vi "bedingungen editor.vi"() -> ()   [LabVIEW 2010]
panel:
  in  "Abfrage Nummer":u32
  in  "löschen":bool
  out "Array":string[][](array[string])
  in  "Stopp":bool
  in  "Abfrage übernehmen":bool
  in  "WertC\n---------------------\nSchreibweise: 0,0042\nT=True; F=False":string
  in  "VariableC":string(combo)
  in  "WertA\n---------------------\nSchreibweise: 0,0042\nT=True; F=False\n---=ungültig":string
  in  "VariableB":string(combo)
  in  "Vergleichsoperator":string(combo)
  in  "VariableA":string(combo)
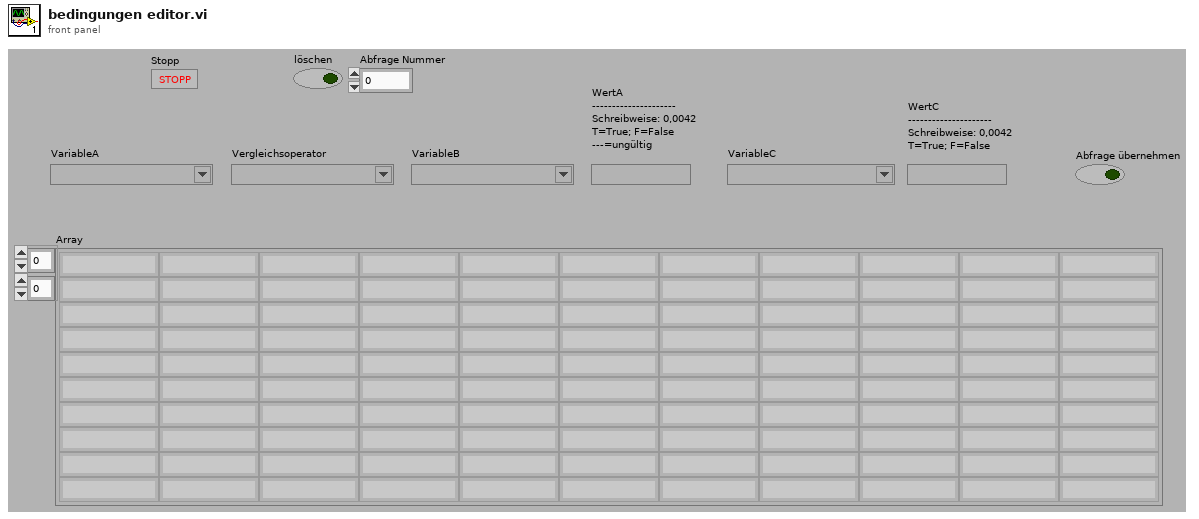
[diagram p1: front panel]
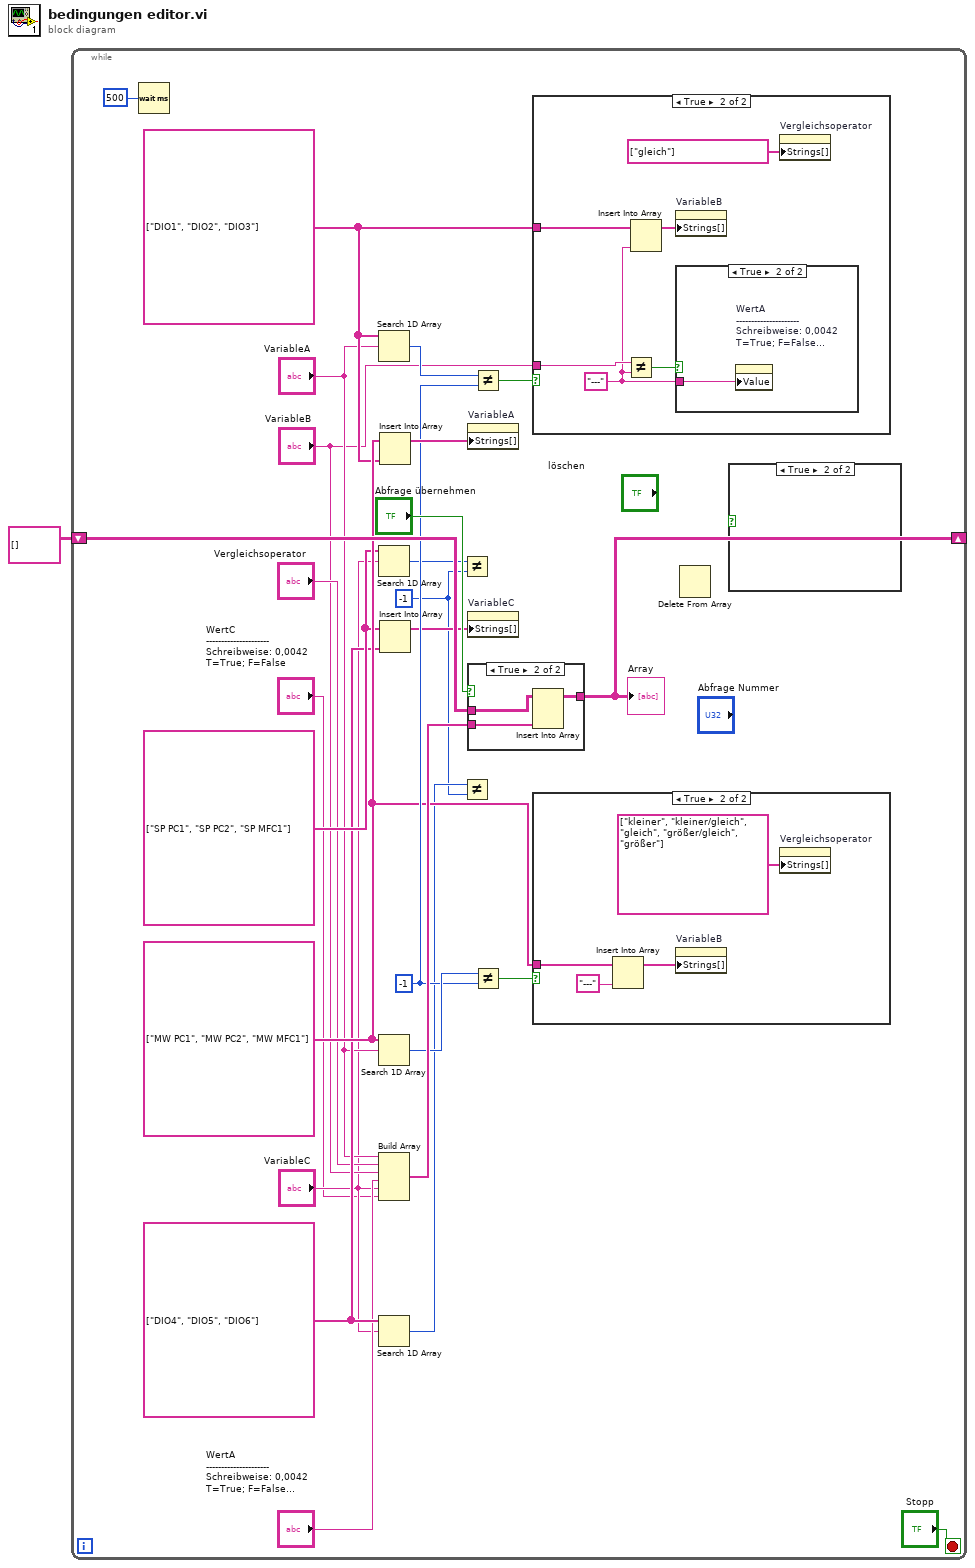
[diagram p0: block diagram]
diagram:
  n1 = while {
    shift-right: [w23] -> _
    shift-left: string[][] [] -> [w24]
    stop <- "Stopp" stop-if-true
    w8 = -1 ("y")
    w10 = string[] ["DIO4", "DIO5", "DIO6"] ("Strings []")
    w12 = string[] ["SP PC1", "SP PC2", "SP MFC1"] ("Strings []")
    w18 = -1 ("y")
    w14 = string[] ["DIO1", "DIO2", "DIO3"] ("Strings []")
    w15 = string[] ["MW PC1", "MW PC2", "MW MFC1"] ("Strings []")
    n2 = Wait (ms)(milliseconds to wait=u32 500 ("Zu wartende ms")) -> ()  [unwired: 1 out]
    n3 = Search 1D Array(1D array=w14, element="VariableA") -> (index of element=w19:i32)  [unwired: 1 in]
    n4 = Search 1D Array(1D array=w12, element="VariableC") -> (index of element=w11:i32)  [unwired: 1 in]
    n5 = Search 1D Array(1D array=w15, element="VariableA") -> (index of element=w20:i32)  [unwired: 1 in]
    n6 = Build Array("VariableA", "Vergleichsoperator", "VariableB", "WertA\n---------------------\nSchreibweise: 0,0042\nT=True; F=False\n---=ungültig", "VariableC", "WertC\n---------------------\nSchreibweise: 0,0042\nT=True; F=False") -> (w25:string[])
    n7 = Search 1D Array(1D array=w10, element="VariableC") -> (index of element=w9:i32)  [unwired: 1 in]
    n8 = Insert Into Array(array=w15, new element=w14) -> (w21:string[])  [unwired: 1 in]
    n9 = Insert Into Array(array=w12, new element=w10) -> (w13:string[])  [unwired: 1 in]
    n10 = Not Equal?(x=w11, y=w8) -> ()  [unwired: 1 out]
    n11 = Not Equal?(x=w9, y=w8) -> ()  [unwired: 1 out]
    n12 = property on="VariableA" class="KombiFeld"("Strings[]"=w21) -> ()  [unwired: 2 in, 2 out]
    n13 = property on="VariableC" class="KombiFeld"("Strings[]"=w13) -> ()  [unwired: 2 in, 2 out]
    n14 = case shown="True" "Abfrage übernehmen" {
      tunnel: w25 -> [_ w41]
      tunnel: w24 -> [w39 w42]
      tunnel: [w39 w40] -> w23
      frame False {
      }
      frame True {
        n15 = Insert Into Array(array=w42, new element=w41) -> (w40:string[][])  [unwired: 2 in]
      }
    }
    "Array" <- w23
    n16 = Not Equal?(x=w19, y=w18) -> (x != y?=w16:bool)
    n17 = Not Equal?(x=w20, y=w18) -> (x != y?=w17:bool)
    n18 = case shown="True" w16 {
      tunnel: w14 -> [_ w32]
      tunnel: "VariableB" -> [_ w30]
      frame False {
      }
      frame True {
        w28 = "---" ("Neues Element/Teil-Array")
        n19 = Not Equal?(x=w30, y=w28) -> (x != y?=w29:bool)
        n20 = Insert Into Array(array=w32, new element=w28) -> (w31:string[])  [unwired: 1 in]
        n21 = property on="VariableB" class="KombiFeld"("Strings[]"=w31) -> ()  [unwired: 2 in, 2 out]
        n22 = case shown="True" w29 {
          tunnel: w28 -> [_ w34]
          frame False {
          }
          frame True {
            n23 = property on="WertA\n---------------------\nSchreibweise: 0,0042\nT=True; F=False\n---=ungültig" class="Str"("Value"=w34) -> ()  [unwired: 2 in, 2 out]
          }
        }
        n24 = property on="Vergleichsoperator" class="KombiFeld"("Strings[]"=string[] ["gleich"] ("Strings []")) -> ()  [unwired: 2 in, 2 out]
      }
    }
    n25 = case shown="True" w17 {
      tunnel: w15 -> [_ w37]
      frame False {
      }
      frame True {
        n26 = Insert Into Array(array=w37, new element="---" ("Neues Element/Teil-Array")) -> (w36:string[])  [unwired: 1 in]
        n27 = property on="VariableB" class="KombiFeld"("Strings[]"=w36) -> ()  [unwired: 2 in, 2 out]
        n28 = property on="Vergleichsoperator" class="KombiFeld"("Strings[]"=string[] ["kleiner", "kleiner/gleich", "gleich", "größer/gleich", "größer"] ("Strings []")) -> ()  [unwired: 2 in, 2 out]
      }
    }
    n29 = Delete From Array() -> ()  [unwired: 3 in, 2 out]
    n30 = case shown="True" {
      selector: _ -> [_ _]
      frame False {
      }
      frame True {
      }
    }
  }
